vi "BotSpeak_LoadScript.vi"(2 "URAPI Script":T2={"Script"="", "Whiles"=[], "Ifs"=[], "Supress Err"=TRUE, "Errors"=""}, 3 "Bot Settings":T1) -> (0 "total response":string="169.254.32.85", 1 "Bot Settings":T1)   [LabVIEW 2012]
doc: "Loads scripted code to the hardware. Will not run without a separate Run VI."
uses:
  <userlib>/botspeak/VIs/Direct/URAPI_Control.ctl
  <userlib>/botspeak/VIs/Direct/BotSpeak_Control.ctl
panel:
  out "SubsString":string
  out "Var Res":string="169.254.32.85"
  out "downloaded fine?":bool
  out "response":string="169.254.32.85"
  out "script":string
  # "Bytes_SIZE = 4\nDIO[3] = 0\nDIO[2] = 1\ncount0=0\n//while0 for 32 iterations\nwhileLand0:\nDIO[3] = 0\nDIO[2] = 0\nDIO[2] = 1\n//end while0 \ncount0+=1\nIF (count0 < 32) goto whileLand0\ncount2=0\n//while2 for 4 iterations\nwhileLand2:\nbyte = Bytes[count2]\ncount4=0\n//while4 for 8 iterations\nwhileLand4:\npulse=byte & 128\npulse = pulse/128\nbyte << = 1\nDIO[3] = pulse\nDIO[2] = 0\nDIO[2] = 1\n//end while4 \ncount4+=1\nIF (count4 < 8) goto whileLand4\n//end while2 \ncount2+=1\nIF (count2 < 4) goto whileLand2\ncount6=0\n//while6 for 32 iterations\nwhileLand6:\nDIO[3] = 0\nDIO[2] = 0\nDIO[2] = 1\n//end while6 \ncount6+=1\nIF (count6 < 32) goto whileLand6\nDIO[2] = 0"
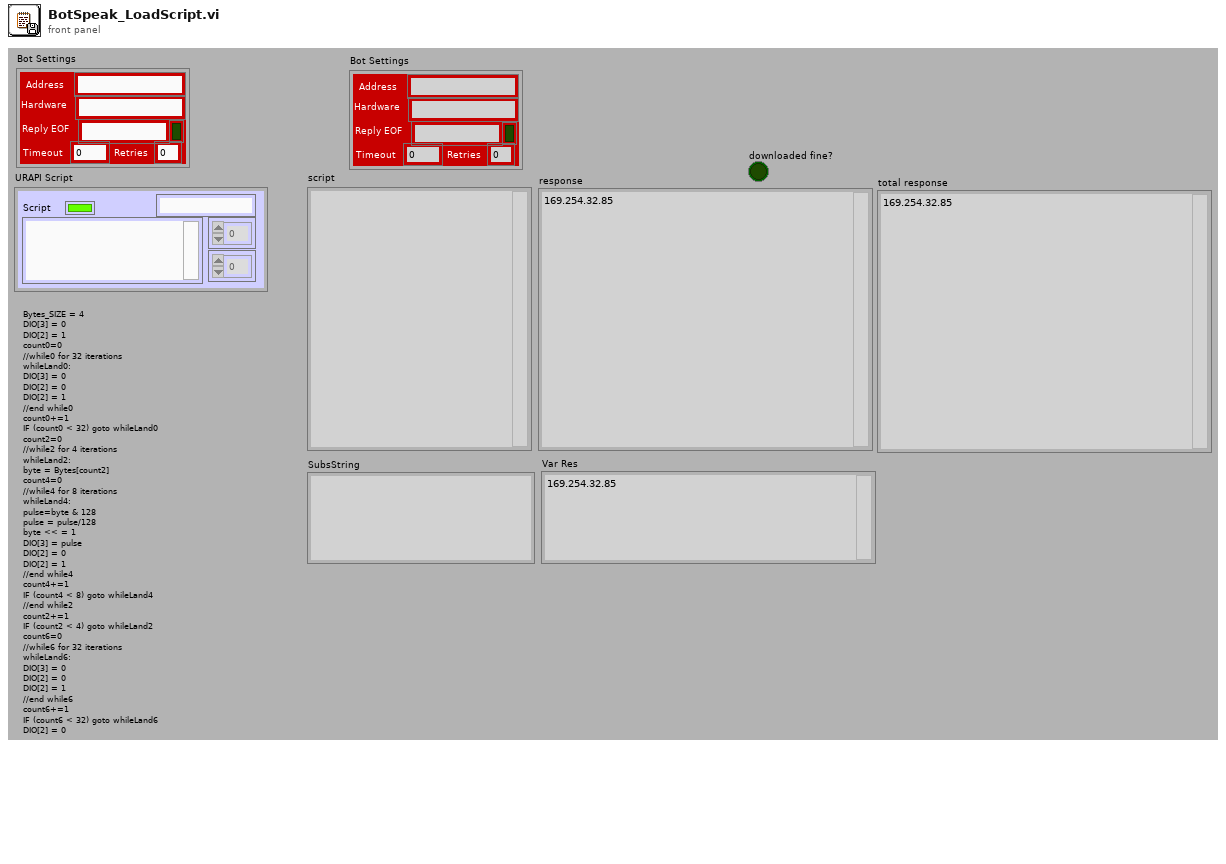
[diagram p1: front panel]
types:
  T1 = typedef "BotSpeak_Control.ctl" = cluster{"Address":string, "Reply EOF":string, "Hardware":string, "Retries":i8, "Timeout":i32, "Open?":bool}
  T2 = typedef "URAPI_Control.ctl" = cluster{"Script":string, "Whiles":u8[], "Ifs":u8[], "Supress Err":bool, "Errors":string}
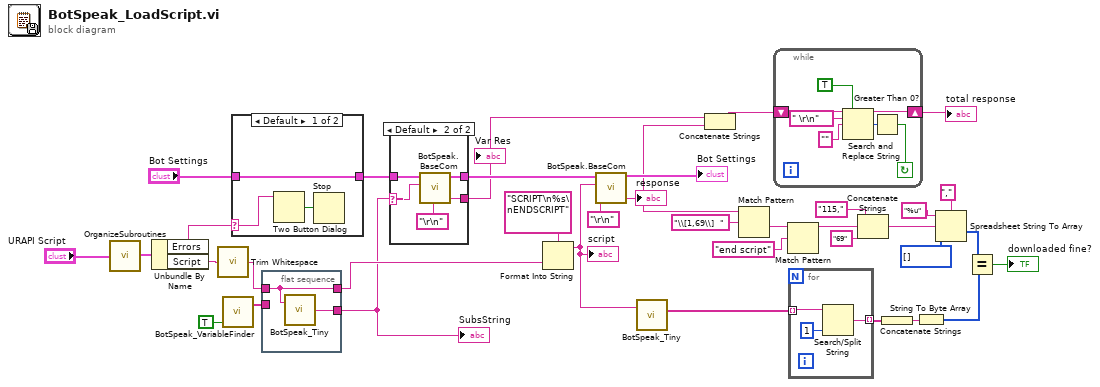
[diagram p0: block diagram]
diagram:
  n1 = call <userlib>:"OrganizeSubroutines.vi"("URAPI Script"="URAPI Script") -> ("URAPI Script"=w15:T2)
  n2 = Unbundle By Name(w15) -> ("Errors"=w18:string, "Script"=w16:string)
  n3 = call <vilib>:"Trim Whitespace.vi"("string"=w16) -> ("trimmed string"=w11:string)  [unwired: 1 in]
  n4 = call <userlib>:"BotSpeak_VariableFinder.vi"("Reset?"=TRUE) -> ("Variables"=w12:string[])  [unwired: 2 in, 1 out]
  n5 = case shown="Default" w18 {
    selector: w18 -> [w38 _]
    tunnel: [w39 w40] -> w7
    tunnel: "Bot Settings" -> [w39 w40]
    frame Default {
      n6 = Two Button Dialog(message=w38) -> (T button?=w37:bool)  [unwired: 2 in]
      n7 = Stop(stop? (T)=w37) -> ()
    }
    frame "" {
    }
  }
  n8 = flat-sequence {
    tunnel: w12 -> [_]
    tunnel: w11 -> [w42]
    tunnel: [w42] -> w10
    tunnel: [w41] -> w3
    frame #0 {
      n9 = call <userlib>:"BotSpeak_Tiny.vi"("URAPI"=w42) -> ("SubsString"=w41:string)  [unwired: 1 in, 2 out]
    }
  }
  n10 = case shown="Default" w3 {
    selector: w3 -> [w43 w45]
    tunnel: w7 -> [w44 w49]
    tunnel: [w44 w48] -> w6
    tunnel: [w43 w47] -> w5
    frame "" {
    }
    frame Default {
      n11 = call <userlib>:"BotSpeak.BaseCom.vi"("Termination"="\r\n", "command"=w45, "Bot Settings in"=w49) -> ("response"=w47:string, "Bot Settings out"=w48:T1)  [unwired: 2 in]
    }
  }
  "Var Res" <- w5
  n12 = Format Into String(format string="SCRIPT\n%s\nENDSCRIPT" ("command"), w10) -> (resulting string=w9:string)  [unwired: 2 in, 1 out]
  "script" <- w9
  n13 = call <userlib>:"BotSpeak.BaseCom.vi"("Termination"="\r\n", "command"=w9, "Bot Settings in"=w6) -> ("response"=w4:string, "Bot Settings out"=→"Bot Settings":T1)  [unwired: 2 in]
  "response" <- w4
  n14 = call <userlib>:"BotSpeak_Tiny.vi"("URAPI"=w9) -> ("Tiny Lines"=w8:string[])  [unwired: 1 in, 2 out]
  n15 = Concatenate Strings(w5, w4) -> (w2:string)
  n16 = Match Pattern(string=w4, regular expression="\\[1,69\\]  ") -> (after substring=w30:string)  [unwired: 1 in, 3 out]
  n17 = while {
    shift-right: [w55] -> w1
    shift-left: w2 -> [w56]
    stop <- w50 continue-if-true
    n18 = Search and Replace String(replace all?=TRUE ("replace all? (F)"), input string=w56, search string=" \r\n", replace string="" ("search string")) -> (result string=w55:string, number of replacements=w51:i32)  [unwired: 4 in, 2 out]
    n19 = Greater Than 0?(x=w51) -> (x > 0?=w50:bool)
  }
  "total response" <- w1
  n20 = Match Pattern(string=w30, regular expression="end script") -> (before substring=w22:string)  [unwired: 1 in, 3 out]
  n21 = for {
    tunnel: w8 -> [w59] mode=indexing
    tunnel: [w57] -> w33 mode=indexing
    n22 = Search/Split String(string=w59, offset (0)=1) -> (match + rest of string=w57:string)  [unwired: 1 in, 2 out]
  }
  n23 = Concatenate Strings("115," ("regular expression"), w22, "69" ("regular expression")) -> (w19:string)
  n24 = Concatenate Strings(w33) -> (w32:string)
  n25 = String To Byte Array(string=w32) -> (unsigned byte array=w25:u8[])
  n26 = Spreadsheet String To Array(delimiter (Tab)=",", format string="%u", spreadsheet string=w19, array type (2D Dbl)=u8[] [] ("unsigned byte array")) -> (array=w24:u8[])
  n27 = Equal?(x=w24, y=w25) -> (x = y?=→"downloaded fine?":bool)
  "SubsString" <- w3
